vi "test_read-nmea-data2.vi"() -> ()   [LabVIEW 2019] (continued)
18,043,,05,37,247,25,06,64,049,25,6*62\n\t\n15:12:12.47\tF9P\t$GPGSV,3,2,09,09,45,074,29,12,23,276,19,17,33,154,23,19,52,157,,6*69\n\t\n15:12:12.49\tF9P\t$GPGSV,3,3,09,25,12,307,,6*5A\n\t\n15:12:12.51\tF9P\t$GLGSV,2,1,08,69,12,031,,70,71,039,28,71,52,205,44,72,04,209,24,1*76\n\t\n15:12:12.53\tF9P\t$GLGSV,2,2,08,77,01,326,,84,20,122,10,85,70,067,37,86,37,330,,1*7D\n\t\n15:12:12.55\tF9P\t$GLGSV,2,1,08,69,12,031,,70,71,039,,71,52,205,22,72,04,209,,3*78\n\t\n15:12:12.57\tF9P\t$GLGSV,2,2,08,77,01,326,,84,20,122,09,85,70,067,20,86,37,330,,3*71\n\t\n15:12:12.59\tF9P\t$GAGSV,2,1,08,02,08,297,10,04,66,117,28,09,32,193,29,11,71,358,28,7*7C\n\t\n15:12:12.61\tF9P\t$GAGSV,2,2,08,12,40,102,28,19,26,045,16,25,09,249,,36,26,308,20,7*76\n\t\n15:12:12.63\tF9P\t$GAGSV,2,1,08,02,08,297,,04,66,117,,09,32,193,,11,71,358,,2*73\n\t\n15:12:12.65\tF9P\t$GAGSV,2,2,08,12,40,102,,19,26,045,,25,09,249,,36,26,308,,2*7C\n\t\n15:12:12.67\tF9P\t$GBGSV,1,1,04,11,50,132,27,14,87,127,24,28,,,22,33,60,219,36,1*49\n\t\n15:12:12.69\tF9P\t$GBGSV,1,1,03,11,50,132,31,14,87,127,31,33,60,219,,3*40\n\t\n15:12:12.71\tF9P\t$GNGLL,3723.53484,N,12656.93169,E,061214.00,A,A*7E\n\t\n15:12:12.73\tF9P\t\t\n15:12:12.75\tF9P\t\t\n15:12:12.77\tF9P\t\t\n15:12:12.79\tF9P\t\t\n15:12:12.81\tF9P\t\t\n15:12:12.83\tF9P\t\t\n15:12:12.85\tF9P\t\t\n15:12:12.87\tF9P\t\t\n15:12:12.89\tF9P\t\t\n15:12:12.91\tF9P\t\t\n15:12:12.93\tF9P\t\t\n15:12:12.95\tF9P\t\t\n15:12:12.97\tF9P\t\t\n15:12:12.99\tF9P\t\t\n15:12:13.01\tF9P\t\t\n15:12:13.03\tF9P\t\t\n15:12:13.05\tF9P\t\t\n15:12:13.07\tF9P\t\t\n15:12:13.09\tF9P\t\t\n15:12:13.11\tF9P\t\t\n15:12:13.13\tF9P\t\t\n15:12:13.15\tF9P\t\t\n15:12:13.17\tF9P\t\t\n15:12:13.19\tF9P\t\t\n15:12:13.21\tF9P\t\t\n15:12:13.23\tF9P\t$GNRMC,061215.00,A,3723.53546,N,12656.93209,E,2.440,28.85,250720,,,A,V*3F\n\t\n15:12:13.25\tF9P\t$GNVTG,28.85,T,,M,2.440,N,4.519,K,A*1F\n\t\n15:12:13.27\tF9P\t$GNGGA,061215.00,3723.53546,N,12656.93209,E,1,12,0.72,38.4,M,18.5,M,,*75\n\t\n15:12:13.29\tF9P\t$GNGSA,A,3,12,06,19,05,17,09,04,02,,,,,1.33,0.72,1.12,1*06\n\t\n15:12:13.31\tF9P\t$GNGSA,A,3,85,70,71,84,,,,,,,,,1.33,0.72,1.12,2*04\n\t\n15:12:13.33\tF9P\t$GNGSA,A,3,36,19,11,04,09,12,,,,,,,1.33,0.72,1.12,3*06\n\t\n15:12:13.35\tF9P\t$GNGSA,A,3,14,11,33,,,,,,,,,,1.33,0.72,1.12,4*07\n\t\n15:12:13.37\tF9P\t$GPGSV,3,1,09,02,55,319,21,04,18,043,22,05,37,247,34,06,64,049,33,1*61\n\t\n15:12:13.39\tF9P\t$GPGSV,3,2,09,09,45,074,31,12,23,276,29,17,33,154,29,19,52,157,32,1*6F\n\t\n15:12:13.41\tF9P\t$GPGSV,3,3,09,25,12,307,12,1*5E\n\t\n15:12:13.43\tF9P\t$GPGSV,3,1,09,02,55,319,,04,18,043,,05,37,247,23,06,64,049,24,6*65\n\t\n15:12:13.45\tF9P\t$GPGSV,3,2,09,09,45,074,27,12,23,276,18,17,33,154,23,19,52,157,,6*66\n\t\n15:12:13.47\tF9P\t$GPGSV,3,3,09,25,12,307,,6*5A\n\t\n15:12:13.49\tF9P\t$GLGSV,2,1,08,69,12,031,,70,71,039,35,71,52,205,41,72,04,209,29,1*72\n\t\n15:12:13.51\tF9P\t$GLGSV,2,2,08,77,01,326,,84,20,122,10,85,70,067,37,86,37,330,,1*7D\n\t\n15:12:13.53\tF9P\t$GLGSV,2,1,08,69,12,031,,70,71,039,,71,52,205,30,72,04,209,,3*7B\n\t\n15:12:13.55\tF9P\t$GLGSV,2,2,08,77,01,326,,84,20,122,12,85,70,067,20,86,37,330,,3*7B\n\t\n15:12:13.57\tF9P\t$GAGSV,2,1,08,02,08,297,08,04,66,117,32,09,32,193,34,11,71,358,29,7*73\n\t\n15:12:13.59\tF9P\t$GAGSV,2,2,08,12,40,102,28,19,26,045,17,25,09,249,,36,26,308,20,7*77\n\t\n15:12:13.61\tF9P\t$GAGSV,2,1,08,02,08,297,,04,66,117,,09,32,193,,11,71,358,,2*73\n\t\n15:12:13.63\tF9P\t$GAGSV,2,2,08,12,40,102,,19,26,045,,25,09,249,,36,26,308,,2*7C\n\t\n15:12:13.65\tF9P\t$GBGSV,1,1,04,11,50,132,32,14,87,127,30,28,,,23,33,60,219,34,1*4B\n\t\n15:12:13.67\tF9P\t$GBGSV,1,1,03,11,50,132,,14,87,127,32,33,60,219,,3*41\n\t\n15:12:13.69\tF9P\t$GNGLL,3723.53546,N,12656.93209,E,061215.00,A,A*75\n\t\n15:12:13.71\tF9P\t\t\n15:12:13.73\tF9P\t\t\n15:12:13.75\tF9P\t\t\n15:12:13.77\tF9P\t\t\n15:12:13.79\tF9P\t\t\n15:12:13.81\tF9P\t\t\n15:12:13.83\tF9P\t\t\n15:12:13.85\tF9P\t\t\n15:12:13.87\tF9P\t\t\n15:12:13.89\tF9P\t\t\n15:12:13.91\tF9P\t\t\n15:12:13.93\tF9P\t\t\n15:12:13.95\tF9P\t\t\n15:12:13.97\tF9P\t\t\n15:12:13.99\tF9P\t\t\n15:12:14.01\tF9P\t\t\n15:12:14.03\tF9P\t\t\n15:12:14.05\tF9P\t\t\n15:12:14.07\tF9P\t\t\n15:12:14.09\tF9P\t\t\n15:12:14.11\tF9P\t\t\n15:12:14.13\tF9P\t\t\n15:12:14.15\tF9P\t\t\n15:12:14.17\tF9P\t\t\n15:12:14.19\tF9P\t\t\n15:12:14.21\tF9P\t\t\n15:12:14.23\tF9P\t$GNRMC,061216.00,A,3723.53588,N,12656.93266,E,2.122,42.04,250720,,,A,V*33\n\t\n15:12:14.25\tF9P\t$GNVTG,42.04,T,,M,2.122,N,3.930,K,A*1B\n\t\n15:12:14.27\tF9P\t$GNGGA,061216.00,3723.53588,N,12656.93266,E,1,12,0.76,38.3,M,18.5,M,,*7E\n\t\n15:12:14.29\tF9P\t$GNGSA,A,3,12,06,19,05,17,09,04,02,,,,,1.35,0.76,1.12,1*04\n\t\n15:12:14.31\tF9P\t$GNGSA,A,3,85,70,71,84,,,,,,,,,1.35,0.76,1.12,2*06\n\t\n15:12:14.33\tF9P\t$GNGSA,A,3,36,19,11,04,09,12,,,,,,,1.35,0.76,1.12,3*04\n\t\n15:12:14.35\tF9P\t$GNGSA,A,3,14,11,33,,,,,,,,,,1.35,0.76,1.12,4*05\n\t\n15:12:14.37\tF9P\t$GPGSV,3,1,09,02,55,319,21,04,18,043,21,05,37,247,31,06,64,049,33,1*67\n\t\n15:12:14.39\tF9P\t$GPGSV,3,2,09,09,45,074,33,12,23,276,27,17,33,154,36,19,52,157,31,1*6E\n\t\n15:12:14.41\tF9P\t$GPGSV,3,3,09,25,12,306,12,1*5F\n\t\n15:12:14.43\tF9P\t$GPGSV,3,1,09,02,55,319,,04,18,043,,05,37,247,25,06,64,049,26,6*61\n\t\n15:12:14.45\tF9P\t$GPGSV,3,2,09,09,45,074,27,12,23,276,19,17,33,154,24,19,52,157,,6*60\n\t\n15:12:14.47\tF9P\t$GPGSV,3,3,09,25,12,306,,6*5B\n\t\n15:12:14.49\tF9P\t$GLGSV,2,1,08,69,12,031,,70,71,039,29,71,52,205,41,72,04,209,27,1*71\n\t\n15:12:14.51\tF9P\t$GLGSV,2,2,08,77,01,326,,84,20,122,09,85,70,067,32,86,37,330,,1*70\n\t\n15:12:14.53\tF9P\t$GLGSV,2,1,08,69,12,031,,70,71,039,,71,52,205,25,72,04,209,,3*7F\n\t\n15:12:14.55\tF9P\t$GLGSV,2,2,08,77,01,326,,84,20,122,12,85,70,067,20,86,37,330,,3*7B\n\t\n15:12:14.57\tF9P\t$GAGSV,2,1,08,02,08,297,07,04,66,117,33,09,32,193,30,11,71,358,31,7*70\n\t\n15:12:14.59\tF9P\t$GAGSV,2,2,08,12,40,102,29,19,26,045,17,25,09,249,,36,26,308,18,7*7D\n\t\n15:12:14.61\tF9P\t$GAGSV,2,1,08,02,08,297,,04,66,117,,09,32,193,32,11,71,358,,2*72\n\t\n15:12:14.63\tF9P\t$GAGSV,2,2,08,12,40,102,,19,26,045,,25,09,249,,36,26,308,,2*7C\n\t\n15:12:14.65\tF9P\t$GBGSV,1,1,04,11,50,132,31,14,87,127,30,28,,,22,33,60,219,31,1*4C\n\t\n15:12:14.67\tF9P\t$GBGSV,1,1,03,11,50,132,,14,87,127,27,33,60,219,,3*45\n\t\n15:12:14.69\tF9P\t$GNGLL,3723.53588,N,12656.93266,E,061216.00,A,A*7D\n\t\n15:12:14.71\tF9P\t\t\n15:12:14.73\tF9P\t\t\n15:12:14.75\tF9P\t\t\n15:12:14.77\tF9P\t\t\n15:12:14.79\tF9P\t\t\n15:12:14.81\tF9P\t\t\n15:12:14.83\tF9P\t\t\n15:12:14.85\tF9P\t\t\n15:12:14.87\tF9P\t\t\n15:12:14.89\tF9P\t\t\n15:12:14.91\tF9P\t\t\n15:12:14.93\tF9P\t\t\n15:12:14.95\tF9P\t\t\n15:12:14.97\tF9P\t\t\n15:12:14.99\tF9P\t\t\n15:12:15.01\tF9P\t\t\n15:12:15.03\tF9P\t\t\n15:12:15.05\tF9P\t\t\n15:12:15.07\tF9P\t\t\n15:12:15.09\tF9P\t\t\n15:12:15.11\tF9P\t\t\n15:12:15.13\tF9P\t\t\n15:12:15.15\tF9P\t\t\n15:12:15.17\tF9P\t\t\n15:12:15.19\tF9P\t\t\n15:12:15.21\tF9P\t\t\n15:12:15.23\tF9P\t\t\n15:12:15.25\tF9P\t$GNRMC,061217.00,A,3723.53632,N,12656.93340,E,2.422,50.03,250720,,,A,V*34\n\t\n15:12:15.27\tF9P\t$GNVTG,50.03,T,,M,2.422,N,4.486,K,A*1D\n\t\n15:12:15.29\tF9P\t$GNGGA,061217.00,3723.53632,N,12656.93340,E,1,12,0.76,38.5,M,18.5,M,,*7E\n\t\n15:12:15.31\tF9P\t$GNGSA,A,3,12,06,19,05,17,09,04,02,,,,,1.35,0.76,1.12,1*04\n\t\n15:12:15.33\tF9P\t$GNGSA,A,3,85,70,71,84,,,,,,,,,1.35,0.76,1.12,2*06\n\t\n15:12:15.35\tF9P\t$GNGSA,A,3,36,19,11,04,09,12,,,,,,,1.35,0.76,1.12,3*04\n\t\n15:12:15.37\tF9P\t$GNGSA,A,3,14,11,33,,,,,,,,,,1.35,0.76,1.12,4*05\n\t\n15:12:15.39\tF9P\t$GPGSV,3,1,09,02,55,319,20,04,18,043,20,05,37,247,31,06,64,049,35,1*61\n\t\n15:12:15.41\tF9P\t$GPGSV,3,2,09,09,45,074,31,12,23,276,26,17,33,154,34,19,52,157,30,1*6E\n\t\n15:12:15.43\tF9P\t$GPGSV,3,3,09,25,12,306,12,1*5F\n\t\n15:12:15.45\tF9P\t$GPGSV,3,1,09,02,55,319,,04,18,043,,05,37,247,25,06,64,049,25,6*62\n\t\n15:12:15.47\tF9P\t$GPGSV,3,2,09,09,45,074,25,12,23,276,19,17,33,154,23,19,52,157,,6*65\n\t\n15:12:15.49\tF9P\t$GPGSV,3,3,09,25,12,306,,6*5B\n\t\n15:12:15.51\tF9P\t$GLGSV,2,1,08,69,12,031,,70,71,039,30,71,52,205,42,72,04,209,27,1*7A\n\t\n15:12:15.53\tF9P\t$GLGSV,2,2,08,77,01,326,,84,20,122,08,85,70,067,42,86,37,330,,1*76\n\t\n15:12:15.55\tF9P\t$GLGSV,2,1,08,69,12,031,,70,71,039,,71,52,205,25,72,04,209,,3*7F\n\t\n15:12:15.57\tF9P\t$GLGSV,2,2,08,77,01,326,,84,20,122,11,85,70,067,20,86,37,330,,3*78\n\t\n15:12:15.59\tF9P\t$GAGSV,2,1,08,02,08,297,09,04,66,117,33,09,32,193,37,11,71,358,34,7*7C\n\t\n15:12:15.61\tF9P\t$GAGSV,2,2,08,12,40,102,33,19,26,045,17,25,09,249,,36,26,308,16,7*78\n\t\n15:12:15.63\tF9P\t$GAGSV,2,1,08,02,08,297,,04,66,117,,09,32,193,,11,71,358,,2*73\n\t\n15:12:15.65\tF9P\t$GAGSV,2,2,08,12,40,102,,19,26,045,,25,09,249,,36,26,308,,2*7C\n\t\n15:12:15.67\tF9P\t$GBGSV,1,1,04,11,50,132,30,14,87,127,23,28,,,21,33,60,219,30,1*4D\n\t\n15:12:15.69\tF9P\t$GBGSV,1,1,03,11,50,132,,14,87,127,28,33,60,219,,3*4A\n\t\n15:12:15.71\tF9P\t$GNGLL,3723.53632,N,12656.93340,E,061217.00,A,A*7B\n\t\n15:12:15.73\tF9P\t\t\n15:12:15.75\tF9P\t\t\n15:12:15.77\tF9P\t\t\n15:12:15.79\tF9P\t\t\n15:12:15.81\tF9P\t\t\n15:12:15.83\tF9P\t\t\n15:12:15.85\tF9P\t\t\n15:12:15.87\tF9P\t\t\n15:12:15.89\tF9P\t\t\n15:12:15.91\tF9P\t\t\n15:12:15.93\tF9P\t\t\n15:12:15.95\tF9P\t\t\n15:12:15.97\tF9P\t\t\n15:12:15.99\tF9P\t\t\n15:12:16.01\tF9P\t\t\n15:12:16.03\tF9P\t\t\n15:12:16.05\tF9P\t\t\n15:12:16.07\tF9P\t\t\n15:12:16.09\tF9P\t\t\n15:12:16.11\tF9P\t\t\n15:12:16.13\tF9P\t\t\n15:12:16.15\tF9P\t\t\n15:12:16.17\tF9P\t\t\n15:12:16.19\tF9P\t\t\n15:12:16.21\tF9P\t\t\n15:12:16.23\tF9P\t\t\n15:12:16.25\tF9P\t$GNRMC,061218.00,A,3723.53705,N,12656.93409,E,2.373,47.75,250720,,,A,V*30\n\t\n15:12:16.27\tF9P\t$GNVTG,47.75,T,,M,2.373,N,4.396,K,A*1F\n\t\n15:12:16.29\tF9P\t$GNGGA,061218.00,3723.53705,N,12656.93409,E,1,12,0.94,36.4,M,18.5,M,,*7D\n\t\n15:12:16.31\tF9P\t$GNGSA,A,3,12,06,19,05,17,09,04,02,,,,,1.65,0.94,1.36,1*0B\n\t\n15:12:16.33\tF9P\t$GNGSA,A,3,85,70,71,84,,,,,,,,,1.65,0.94,1.36,2*09\n\t\n15:12:16.35\tF9P\t$GNGSA,A,3,36,19,11,04,09,12,,,,,,,1.65,0.94,1.36,3*0B\n\t\n15:12:16.37\tF9P\t$GNGSA,A,3,14,11,33,,,,,,,,,,1.65,0.94,1.36,4*0A\n\t\n15:12:16.39\tF9P\t$GPGSV,3,1,09,02,55,319,21,04,18,043,22,05,37,247,30,06,64,049,36,1*60\n\t\n15:12:16.41\tF9P\t$GPGSV,3,2,09,09,45,074,31,12,23,276,27,17,33,154,33,19,52,157,31,1*69\n\t\n15:12:16.43\tF9P\t$GPGSV,3,3,09,25,12,306,12,1*5F\n\t\n15:12:16.45\tF9P\t$GPGSV,3,1,09,02,55,319,,04,18,043,19,05,37,247,25,06,64,049,23,6*6C\n\t\n15:12:16.47\tF9P\t$GPGSV,3,2,09,09,45,074,26,12,23,276,20,17,33,154,30,19,52,157,,6*6E\n\t\n15:12:16.49\tF9P\t$GPGSV,3,3,09,25,12,306,,6*5B\n\t\n15:12:16.51\tF9P\t$GLGSV,2,1,08,69,12,031,,70,71,039,34,71,52,205,44,72,04,209,25,1*7A\n\t\n15:12:16.53\tF9P\t$GLGSV,2,2,08,77,01,326,,84,20,122,09,85,70,067,37,86,37,330,,1*75\n\t\n15:12:16.55\tF9P\t$GLGSV,2,1,08,69,12,031,,70,71,039,,71,52,205,30,72,04,209,,3*7B\n\t\n15:12:16.57\tF9P\t$GLGSV,2,2,08,77,01,326,,84,20,122,14,85,70,067,20,86,37,330,,3*7D\n\t\n15:12:16.59\tF9P\t$GAGSV,2,1,08,02,08,297,08,04,66,117,31,09,32,193,34,11,71,358,36,7*7E\n\t\n15:12:16.61\tF9P\t$GAGSV,2,2,08,12,40,102,30,19,26,045,15,25,09,249,,36,26,308,16,7*79\n\t\n15:12:16.63\tF9P\t$GAGSV,2,1,08,02,08,297,,04,66,117,,09,32,193,,11,71,358,,2*73\n\t\n15:12:16.65\tF9P\t$GAGSV,2,2,08,12,40,102,,19,26,045,,25,09,249,,36,26,308,,2*7C\n\t\n15:12:16.67\tF9P\t$GBGSV,1,1,04,11,50,132,30,14,87,127,30,28,,,21,33,60,219,39,1*46\n\t\n15:12:16.69\tF9P\t$GBGSV,1,1,03,11,50,132,,14,87,127,29,33,60,219,,3*4B\n\t\n15:12:16.71\tF9P\t$GNGLL,3723.53705,N,12656.93409,E,061218.00,A,A*7B\n\t\n15:12:16.73\tF9P\t\t\n15:12:16.75\tF9P\t\t\n15:12:16.77\tF9P\t\t\n15:12:16.79\tF9P\t\t\n15:12:16.81\tF9P\t\t\n15:12:16.83\tF9P\t\t\n15:12:16.85\tF9P\t\t\n15:12:16.87\tF9P\t\t\n15:12:16.89\tF9P\t\t\n15:12:16.91\tF9P\t\t\n15:12:16.93\tF9P\t\t\n15:12:16.95\tF9P\t\t\n15:12:16.97\tF9P\t\t\n15:12:16.99\tF9P\t\t\n15:12:17.01\tF9P\t\t\n15:12:17.03\tF9P\t\t\n15:12:17.05\tF9P\t\t\n15:12:17.07\tF9P\t\t\n15:12:17.09\tF9P\t\t\n15:12:17.11\tF9P\t\t\n15:12:17.13\tF9P\t\t\n15:12:17.15\tF9P\t\t\n15:12:17.17\tF9P\t\t\n15:12:17.19\tF9P\t\t\n15:12:17.21\tF9P\t\t\n15:12:17.23\tF9P\t$GNRMC,061219.00,A,3723.53756,N,12656.93462,E,2.525,38.70,250720,,,A,V*32\n\t\n15:12:17.25\tF9P\t$GNVTG,38.70,T,,M,2.525,N,4.677,K,A*1D\n\t\n15:12:17.27\tF9P\t$GNGGA,061219.00,3723.53756,N,12656.93462,E,1,12,0.76,36.9,M,18.5,M,,*76\n\t\n15:12:17.29\tF9P\t$GNGSA,A,3,12,06,19,05,17,09,04,02,,,,,1.35,0.76,1.12,1*04\n\t\n15:12:17.31\tF9P\t$GNGSA,A,3,85,70,71,84,,,,,,,,,1.35,0.76,1.12,2*06\n\t\n15:12:17.33\tF9P\t$GNGSA,A,3,36,19,11,04,09,12,,,,,,,1.35,0.76,1.12,3*04\n\t\n15:12:17.35\tF9P\t$GNGSA,A,3,14,11,33,,,,,,,,,,1.35,0.76,1.12,4*05\n\t\n15:12:17.37\tF9P\t$GPGSV,3,1,09,02,55,319,21,04,18,043,22,05,37,247,34,06,64,049,29,1*6A\n\t\n15:12:17.39\tF9P\t$GPGSV,3,2,09,09,45,074,27,12,23,276,27,17,33,154,35,19,52,157,31,1*68\n\t\n15:12:17.41\tF9P\t$GPGSV,3,3,09,25,12,306,13,1*5E\n\t\n15:12:17.43\tF9P\t$GPGSV,3,1,09,02,55,319,,04,18,043,16,05,37,247,25,06,64,049,23,6*63\n\t\n15:12:17.45\tF9P\t$GPGSV,3,2,09,09,45,074,25,12,23,276,20,17,33,154,29,19,52,157,,6*65\n\t\n15:12:17.47\tF9P\t$GPGSV,3,3,09,25,12,306,,6*5B\n\t\n15:12:17.49\tF9P\t$GLGSV,2,1,08,69,12,031,,70,71,039,23,71,52,205,45,72,04,209,26,1*7E\n\t\n15:12:17.51\tF9P\t$GLGSV,2,2,08,77,01,326,,84,20,122,11,85,70,067,36,86,37,330,,1*7D\n\t\n15:12:17.53\tF9P\t$GLGSV,2,1,08,69,12,031,,70,71,039,,71,52,205,29,72,04,209,,3*73\n\t\n15:12:17.55\tF9P\t$GLGSV,2,2,08,77,01,326,,84,20,122,15,85,70,067,21,86,37,330,,3*7D\n\t\n15:12:17.57\tF9P\t$GAGSV,2,1,08,02,08,297,10,04,66,117,31,09,32,193,34,11,71,358,28,7*78\n\t\n15:12:17.59\tF9P\t$GAGSV,2,2,08,12,40,102,30,19,26,045,14,25,09,249,,36,26,308,18,7*76\n\t\n15:12:17.61\tF9P\t$GAGSV,2,1,08,02,08,297,,04,66,117,,09,32,193,,11,71,358,,2*73\n\t\n15:12:17.63\tF9P\t$GAGSV,2,2,08,12,40,102,,19,26,045,,25,09,249,,36,26,308,,2*7C\n\t\n15:12:17.65\tF9P\t$GBGSV,1,1,04,11,50,132,30,14,87,127,30,28,,,21,33,60,219,35,1*4A\n\t\n15:12:17.67\tF9P\t$GBGSV,1,1,03,11,50,132,25,14,87,127,33,33,60,219,,3*47\n\t\n15:12:17.69\tF9P\t$GNGLL,3723.53756,N,12656.93462,E,061219.00,A,A*71\n\t\n15:12:17.71\tF9P\t\t\n15:12:17.73\tF9P\t\t\n15:12:17.75\tF9P\t\t\n15:12:17.77\tF9P\t\t\n15:12:17.79\tF9P\t\t\n15:12:17.81\tF9P\t\t\n15:12:17.83\tF9P\t\t\n15:12:17.85\tF9P\t\t\n15:12:17.87\tF9P\t\t\n15:12:17.89\tF9P\t\t\n15:12:17.91\tF9P\t\t\n15:12:17.93\tF9P\t\t\n15:12:17.95\tF9P\t\t\n15:12:17.97\tF9P\t\t\n15:12:17.99\tF9P\t\t\n15:12:18.01\tF9P\t\t\n15:12:18.03\tF9P\t\t\n15:12:18.05\tF9P\t\t\n15:12:18.07\tF9P\t\t\n15:12:18.09\tF9P\t\t\n15:12:18.11\tF9P\t\t\n15:12:18.13\tF9P\t\t\n15:12:18.15\tF9P\t\t\n15:12:18.17\tF9P\t\t\n15:12:18.19\tF9P\t\t\n15:12:18.21\tF9P\t\t\n15:12:18.23\tF9P\t$GNRMC,061220.00,A,3723.53810,N,12656.93538,E,2.965,37.10,250720,,,A,V*3A\n\t\n15:12:18.25\tF9P\t$GNVTG,37.10,T,,M,2.965,N,5.492,K,A*14\n\t\n15:12:18.27\tF9P\t$GNGGA,061220.00,3723.53810,N,12656.93538,E,1,12,0.76,37.9,M,18.5,M,,*7E\n\t\n15:12:18.29\tF9P\t$GNGSA,A,3,12,06,19,05,17,09,04,02,,,,,1.35,0.76,1.12,1*04\n\t\n15:12:18.31\tF9P\t$GNGSA,A,3,85,70,71,84,,,,,,,,,1.35,0.76,1.12,2*06\n\t\n15:12:18.33\tF9P\t$GNGSA,A,3,36,19,11,04,09,12,,,,,,,1.35,0.76,1.12,3*04\n\t\n15:12:18.35\tF9P\t$GNGSA,A,3,14,11,33,,,,,,,,,,1.35,0.76,1.12,4*05\n\t\n15:12:18.37\tF9P\t$GPGSV,3,1,09,02,55,319,21,04,18,043,22,05,37,247,37,06,64,049,29,1*69\n\t\n15:12:18.39\tF9P\t$GPGSV,3,2,09,09,45,074,32,12,23,276,31,17,33,154,36,19,52,157,31,1*68\n\t\n15:12:18.41\tF9P\t$GPGSV,3,3,09,25,12,306,14,1*59\n\t\n15:12:18.43\tF9P\t$GPGSV,3,1,09,02,55,319,,04,18,043,15,05,37,247,25,06,64,049,23,6*60\n\t\n15:12:18.45\tF9P\t$GPGSV,3,2,09,09,45,074,27,12,23,276,21,17,33,154,27,19,52,157,,6*68\n\t\n15:12:18.47\tF9P\t$GPGSV,3,3,09,25,12,306,,6*5B\n\t\n15:12:18.49\tF9P\t$GLGSV,2,1,08,69,12,031,,70,71,039,30,71,52,205,38,72,04,209,26,1*76\n\t\n15:12:18.51\tF9P\t$GLGSV,2,2,08,77,01,326,,84,20,122,11,85,70,067,40,86,37,330,,1*7C\n\t\n15:12:18.53\tF9P\t$GLGSV,2,1,08,69,12,031,,70,71,039,,71,52,205,28,72,04,209,,3*72\n\t\n15:12:18.55\tF9P\t$GLGSV,2,2,08,77,01,326,,84,20,122,16,85,70,067,22,86,37,330,,3*7D\n\t\n15:12:18.57\tF9P\t$GAGSV,2,1,08,02,08,297,09,04,66,117,31,09,32,193,33,11,71,358,27,7*78\n\t\n15:12:18.59\tF9P\t$GAGSV,2,2,08,12,40,102,33,19,26,045,14,25,09,249,,36,26,308,17,7*7A\n\t\n15:12:18.61\tF9P\t$GAGSV,2,1,08,02,08,297,,04,66,117,,09,32,193,,11,71,358,,2*73\n\t\n15:12:18.63\tF9P\t$GAGSV,2,2,08,12,40,102,,19,26,045,,25,09,249,,36,26,308,,2*7C\n\t\n15:12:18.65\tF9P\t$GBGSV,1,1,04,11,50,132,27,14,87,127,24,28,,,21,33,60,219,27,1*4A\n\t\n15:12:18.67\tF9P\t$GBGSV,1,1,03,11,50,132,,14,87,127,29,33,60,219,,3*4B\n\t\n15:12:18.69\tF9P\t$GNGLL,3723.53810,N,12656.93538,E,061220.00,A,A*78\n\t\n15:12:18.71\tF9P\t\t\n15:12:18.73\tF9P\t\t\n15:12:18.75\tF9P\t\t\n15:12:18.77\tF9P\t\t\n15:12:18.79\tF9P\t\t\n15:12:18.81\tF9P\t\t\n15:12:18.83\tF9P\t\t\n15:12:18.85\tF9P\t\t\n15:12:18.87\tF9P\t\t\n15:12:18.89\tF9P\t\t\n15:12:18.91\tF9P\t\t\n15:12:18.93\tF9P\t\t\n15:12:18.95\tF9P\t\t\n15:12:18.97\tF9P\t\t\n15:12:18.99\tF9P\t\t\n15:12:19.01\tF9P\t\t\n15:12:19.03\tF9P\t\t\n15:12:19.05\tF9P\t\t\n15:12:19.07\tF9P\t\t\n15:12:19.09\tF9P\t\t\n15:12:19.11\tF9P\t\t\n15:12:19.13\tF9P\t\t\n15:12:19.15\tF9P\t\t\n15:12:19.17\tF9P\t\t\n15:12:19.19\tF9P\t\t\n15:12:19.21\tF9P\t\t\n15:12:19.23\tF9P\t\t\n15:12:19.25\tF9P\t$GNRMC,061221.00,A,3723.53846,N,12656.93612,E,2.351,41.93,250720,,,A,V*34\n\t\n15:12:19.27\tF9P\t$GNVTG,41.93,T,,M,2.351,N,4.353,K,A*18\n\t\n15:12:19.29\tF9P\t$GNGGA,061221.00,3723.53846,N,12656.93612,E,1,12,0.73,39.4,M,18.5,M,,*71\n\t\n15:12:19.31\tF9P\t$GNGSA,A,3,12,06,19,05,17,09,04,02,,,,,1.26,0.73,1.03,1*03\n\t\n15:12:19.33\tF9P\t$GNGSA,A,3,85,70,71,84,,,,,,,,,1.26,0.73,1.03,2*01\n\t\n15:12:19.35\tF9P\t$GNGSA,A,3,36,19,11,04,09,12,,,,,,,1.26,0.73,1.03,3*03\n\t\n15:12:19.37\tF9P\t$GNGSA,A,3,14,11,33,,,,,,,,,,1.26,0.73,1.03,4*02\n\t\n15:12:19.39\tF9P\t$GPGSV,3,1,09,02,55,319,20,04,18,043,23,05,37,247,32,06,64,049,36,1*62\n\t\n15:12:19.41\tF9P\t$GPGSV,3,2,09,09,45,074,32,12,23,276,31,17,33,154,29,19,52,157,30,1*67\n\t\n15:12:19.43\tF9P\t$GPGSV,3,3,09,25,12,306,13,1*5E\n\t\n15:12:19.45\tF9P\t$GPGSV,3,1,09,02,55,319,,04,18,043,27,05,37,247,25,06,64,049,25,6*67\n\t\n15:12:19.47\tF9P\t$GPGSV,3,2,09,09,45,074,26,12,23,276,21,17,33,154,27,19,52,157,,6*69\n\t\n15:12:19.49\tF9P\t$GPGSV,3,3,09,25,12,306,,6*5B\n\t\n15:12:19.51\tF9P\t$GLGSV,2,1,08,69,12,031,,70,71,039,32,71,52,205,37,72,04,209,26,1*7B\n\t\n15:12:19.53\tF9P\t$GLGSV,2,2,08,77,01,326,,84,20,122,09,85,70,067,36,86,37,330,,1*74\n\t\n15:12:19.55\tF9P\t$GLGSV,2,1,08,69,12,031,,70,71,039,,71,52,205,26,72,04,209,,3*7C\n\t\n15:12:19.57\tF9P\t$GLGSV,2,2,08,77,01,326,,84,20,122,16,85,70,067,23,86,37,330,,3*7C\n\t\n15:12:19.59\tF9P\t$GAGSV,2,1,08,02,08,297,07,04,66,117,30,09,32,193,30,11,71,358,37,7*75\n\t\n15:12:19.61\tF9P\t$GAGSV,2,2,08,12,40,102,29,19,26,045,14,25,09,249,,36,26,308,16,7*70\n\t\n15:12:19.63\tF9P\t$GAGSV,2,1,08,02,08,297,,04,66,117,,09,32,193,,11,71,358,,2*73\n\t\n15:12:19.65\tF9P\t$GAGSV,2,2,08,12,40,102,,19,26,045,,25,09,249,,36,26,308,,2*7C\n\t\n15:12:19.67\tF9P\t$GBGSV,1,1,04,11,50,132,28,14,87,127,30,28,,,19,33,60,219,29,1*45\n\t\n15:12:19.69\tF9P\t$GBGSV,1,1,03,11,50,132,33,14,87,127,29,33,60,219,,3*4B\n\t\n15:12:19.71\tF9P\t$GNGLL,3723.53846,N,12656.93612,E,061221.00,A,A*71\n\t\n15:12:19.73\tF9P\t\t\n15:12:19.75\tF9P\t\t\n15:12:19.77\tF9P\t\t\n15:12:19.79\tF9P\t\t\n15:12:19.81\tF9P\t\t\n15:12:19.83\tF9P\t\t\n15:12:19.85\tF9P\t\t\n15:12:19.87\tF9P\t\t\n15:12:19.89\tF9P\t\t\n15:12:19.91\tF9P\t\t\n15:12:19.93\tF9P\t\t\n15:12:19.95\tF9P\t\t\n15:12:19.97\tF9P\t\t\n15:12:19.99\tF9P\t\t\n15:12:20.01\tF9P\t\t\n15:12:20.03\tF9P\t\t\n15:12:20.05\tF9P\t\t\n15:12:20.07\tF9P\t\t\n15:12:20.09\tF9P\t\t\n15:12:20.11\tF9P\t\t\n15:12:20.13\tF9P\t\t\n15:12:20.15\tF9P\t\t\n15:12:20.17\tF9P\t\t\n15:12:20.19\tF9P\t\t\n15:12:20.21\tF9P\t\t\n15:12:20.23\tF9P\t\t\n15:12:20.25\tF9P\t$GNRMC,061222.00,A,3723.53875,N,12656.93680,E,2.455,57.59,250720,,,A,V*3E\n\t\n15:12:20.27\tF9P\t$GNVTG,57.59,T,,M,2.455,N,4.546,K,A*18\n\t\n15:12:20.29\tF9P\t$GNGGA,061222.00,3723.53875,N,12656.93680,E,1,12,0.73,40.7,M,18.5,M,,*74\n\t\n15:12:20.31\tF9P\t$GNGSA,A,
